vi "Callsign.vi"() -> ()   [LabVIEW 2020]
panel:
  out "unsigned byte array":u8[](array[numeric]) format="%08b"
  out "Array":string[](array[string])
  out "Callsign":string
  out "Type ID Binary":u8 format="%08b"
  out "Format Binary":u8 format="%08b"
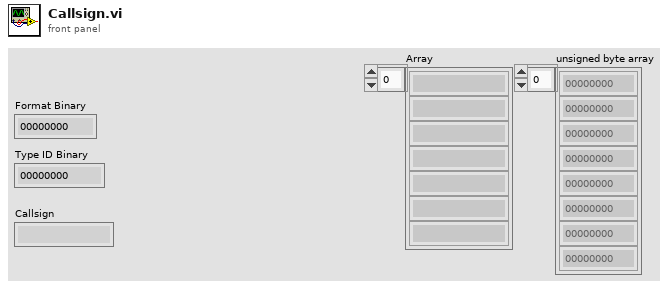
[diagram p1: front panel]
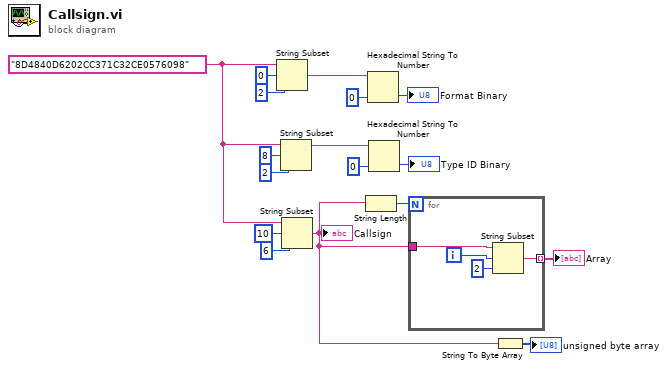
[diagram p0: block diagram]
diagram:
  w5 = "8D4840D6202CC371C32CE0576098"
  n1 = String Subset(string=w5, offset (0)=0, length (rest)=2 ("length (rest)")) -> (substring=w13:string)
  n2 = String Subset(string=w5, offset (0)=8, length (rest)=2 ("length (rest)")) -> (substring=w8:string)
  n3 = String Subset(string=w5, offset (0)=10, length (rest)=6 ("length (rest)")) -> (substring=w2:string)
  "Callsign" <- w2
  n4 = String Length(string=w2) -> (length=w4:i32)
  n5 = Hexadecimal String To Number(string=w13, default (0uL)=u8 0 ("default (0 U32)")) -> (number=→"Format Binary":u8)  [unwired: 1 in, 1 out]
  n6 = Hexadecimal String To Number(string=w8, default (0uL)=u8 0 ("default (0 U32)")) -> (number=→"Type ID Binary":u8)  [unwired: 1 in, 1 out]
  n7 = for {
    N: w4 -> [_]
    tunnel: w2 -> [w21]
    tunnel: [w18] -> w3 mode=indexing
    i -> [w20]
    n8 = String Subset(string=w21, offset (0)=w20, length (rest)=2 ("length (rest)")) -> (substring=w18:string)
  }
  "Array" <- w3
  n9 = String To Byte Array(string=w2) -> (unsigned byte array=→"unsigned byte array":u8[])
